vi "Write_Status.vi"(6 "Error In":errorcluster, 8 "Tea Powder\n       (Kg)":u32(slide) scale=0.0..10000.0, 9 "Coffee Powder\n         (Kg)":u32(slide) scale=0.0..10000.0, 10 "Water\n   (Lt)":u32(slide) scale=0.0..10000.0, 11 "Milk\n (Lt)":u32(slide) scale=0.0..10000.0) -> (0 "Error Out":errorcluster)   [LabVIEW 2014]
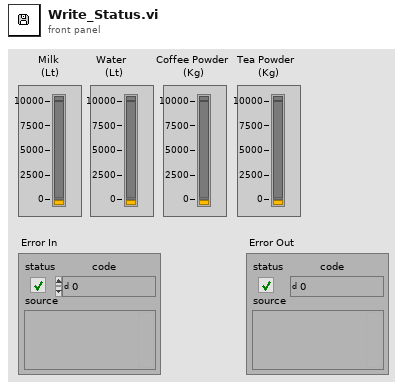
[diagram p1: front panel]
types:
  T1 = enum16{"open", "replace", "create", "open or create", "replace or create", "replace or create with confirmation"}
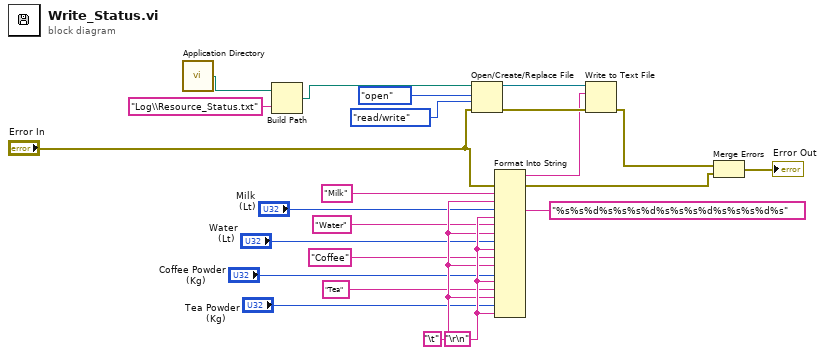
[diagram p0: block diagram]
diagram:
  w16 = "\r\n"
  w15 = "\t"
  n1 = call <vilib>:"Application Directory.vi"() -> ("Application Directory"=w22:path)
  n2 = Build Path(base path=w22, name or relative path="Log\\Resource_Status.txt") -> (appended path=w21:path)
  n3 = Open/Create/Replace File(file path (use dialog)=w21, error in="Error In", operation (0:open)=T1."open", access (0:read/write)=enum16{"read/write", "read-only", "write-only"}."read/write") -> (refnum out=w18:refnum<file>, error out=w6:errorcluster)  [unwired: 2 in, 1 out]
  n4 = Format Into String "Format Into String"(format string="%s%s%d%s%s%s%d%s%s%s%d%s%s%s%d%s", error in="Error In", "Milk" ("input 1"), w15, "Milk\n (Lt)", w16, "Water" ("input 1"), w15, "Water\n   (Lt)", w16, "Coffee" ("input 1"), w15, "Coffee Powder\n         (Kg)", w16, "Tea" ("input 1"), w15, "Tea Powder\n       (Kg)", w16) -> (resulting string=w5:string, error out=w2:errorcluster)  [unwired: 1 in]
  n5 = Write to Text File(file (use dialog)=w18, text=w5, error in=w6) -> (error out=w3:errorcluster)  [unwired: 1 in, 2 out]
  n6 = Merge Errors "Merge Errors"(w3, w2) -> (→"Error Out":errorcluster)
